vi "写入当前获取数据.vi"(8 "error in (no error)":errorcluster caption="错误输入（无错误）", 11 "抽取参数输入":refnum<class "抽取参数.lvclass">) -> (0 "error out":errorcluster caption="错误输出", 3 "抽取参数输出":refnum<class "抽取参数.lvclass">)   [LabVIEW 2020, in "抽取参数.lvclass"]
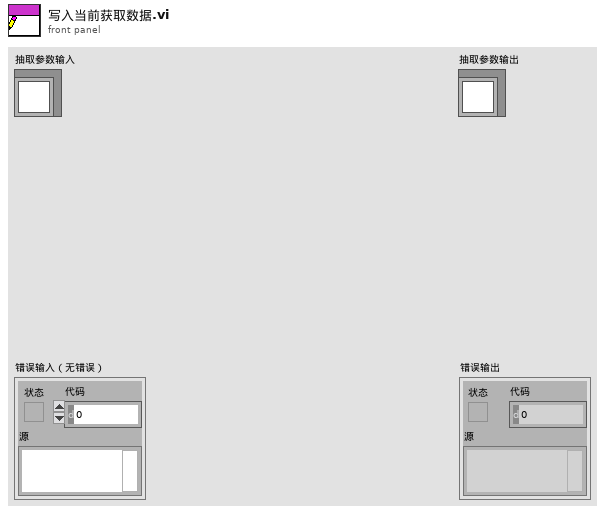
[diagram p1: front panel]
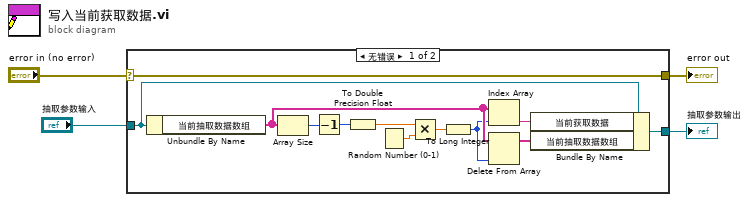
[diagram p0: block diagram]
diagram:
  n1 = case shown="无错误" "error in (no error)" {
    selector: "error in (no error)" -> [w16 w17]
    tunnel: [w16 w17] -> w3
    tunnel: [w15 w18] -> w1
    tunnel: "抽取参数输入" -> [w14 w18]
    frame No Error {
      n2 = Unbundle By Name(w14) -> ("当前抽取数据数组"=w8:string[])
      n3 = Array Size(array=w8) -> (size(s)=w13:i32)
      n4 = Decrement(x=w13) -> (x-1=w12:i32)
      n5 = To Double Precision Float(number=w12) -> (double precision float=w11:dbl)
      n6 = Random Number (0-1)() -> (number: 0 to 1=w10:dbl)
      n7 = Multiply(x=w11, y=w10) -> (x*y=w9:dbl)
      n8 = To Long Integer(number=w9) -> (32bit integer=w7:i32)
      n9 = Index Array(array=w8, index=w7) -> (element=w5:string)
      n10 = Delete From Array(array=w8, index=w7) -> (array with subset deleted=w6:string[])  [unwired: 1 in, 1 out]
      n11 = Bundle By Name(cluster=w14, "当前获取数据"=w5, "当前抽取数据数组"=w6) -> (w15:refnum<class "抽取参数.lvclass">)
    }
    frame Error {
    }
  }
  "error out" <- w3
  "抽取参数输出" <- w1
